vi "LensAndCameraCalibration-GFV.vi"(8 "error in (no error)":errorcluster, 10 "Variant In":variant, 11 "LensCalibrationCtl":T1=enum."Get Calibration") -> (0 "error out":errorcluster, 3 "Variant Out":variant)   [LabVIEW 2015]
doc: "Use this template to build a VI to use as a subVI."
uses:
  LensCalibrationCtlGFV.ctl
  LensCalibrationModel.ctl
  <vilib>/Utility/file.llb/Read From Spreadsheet File (string).vi
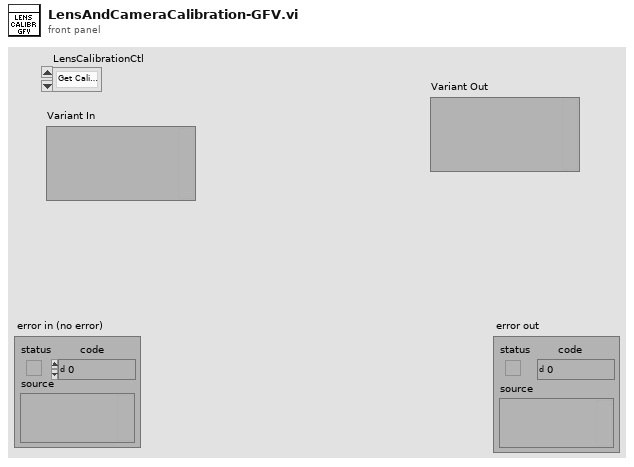
[diagram p1: front panel]
types:
  T1 = typedef "LensCalibrationCtlGFV.ctl" = enum16{"Get MicronPerPixel", "Get Range and PixelsForRange", "Get Mag Names", "Get Calibration", "Read Calibration From File", "Init"}
  T2 = cluster{"MagRingText":u16, "High Resolution":bool}
  T3 = typedef "LensCalibrationModel.ctl" = cluster{"Lens Mag":string, "MicronsPerPixels":dbl, "Scale in microns":i32, "High Resolution":bool}[]
  T4 = cluster{"Lens Mag":string, "MicronsPerPixels":dbl, "Scale in microns":i32, "High Resolution":bool}
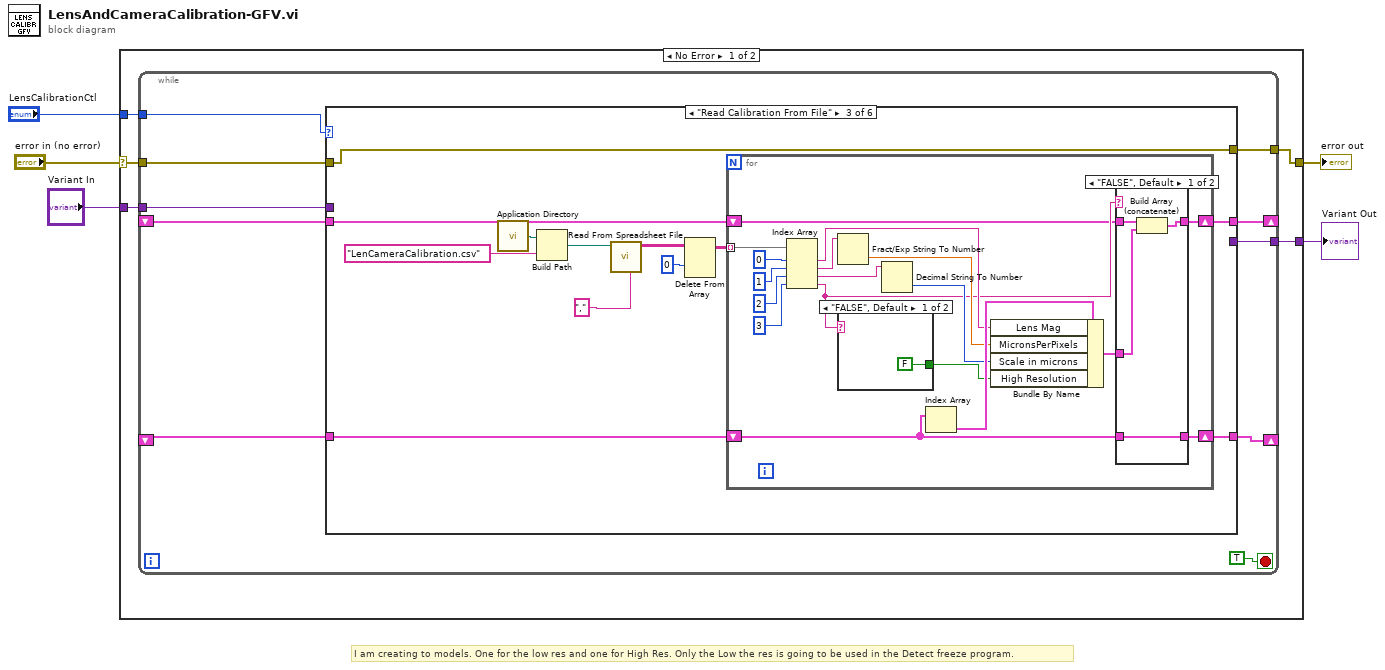
[diagram p0: block diagram]
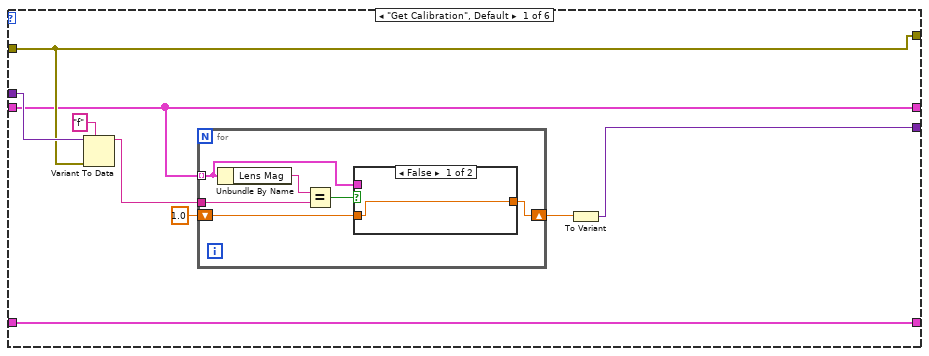
[diagram p2: hidden frame]
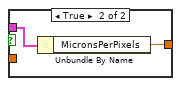
[diagram p3: hidden frame]
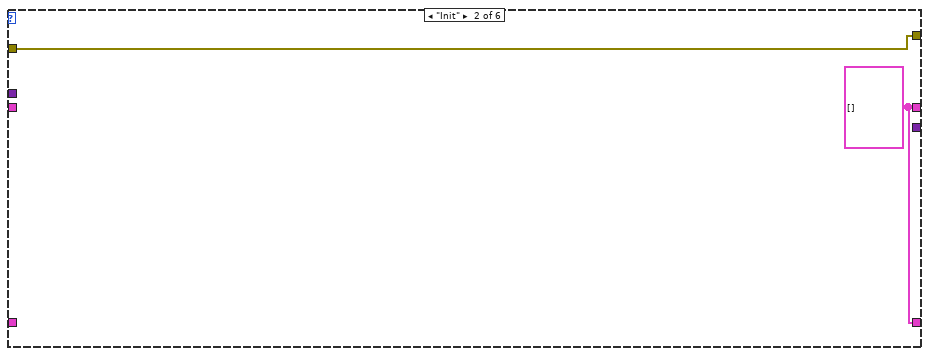
[diagram p4: hidden frame]
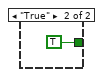
[diagram p5: hidden frame]
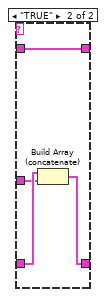
[diagram p6: hidden frame]
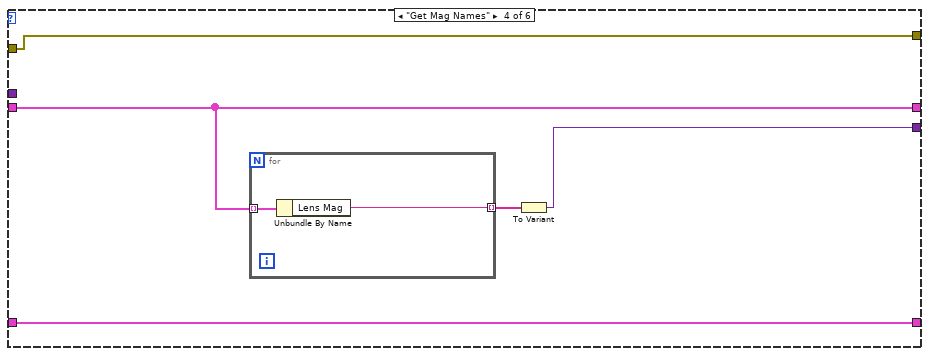
[diagram p7: hidden frame]
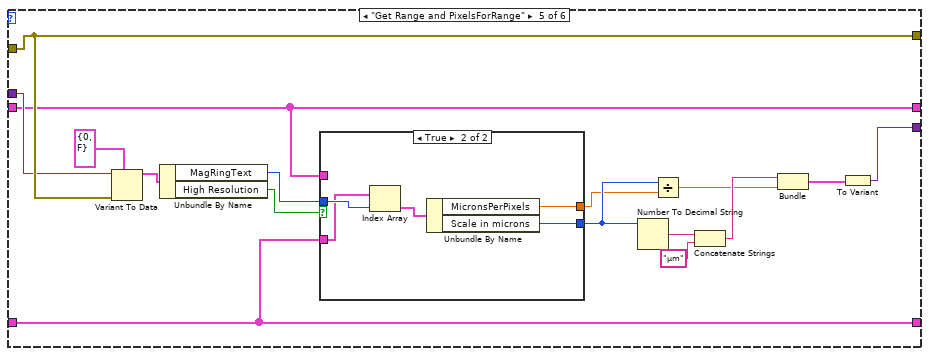
[diagram p8: hidden frame]
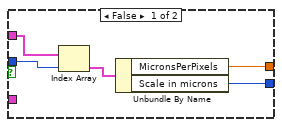
[diagram p9: hidden frame]
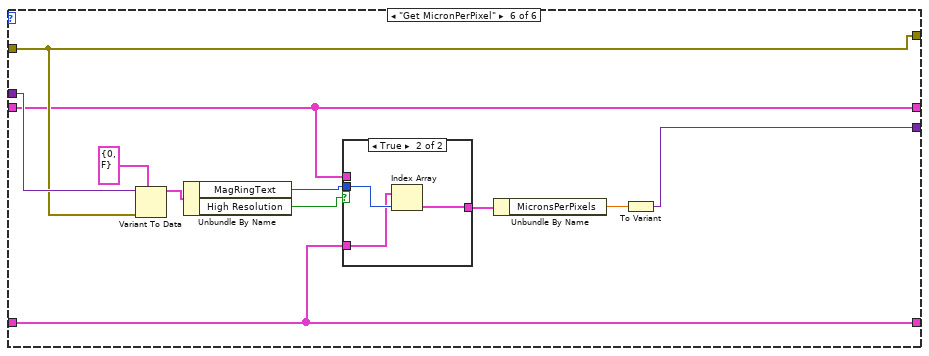
[diagram p10: hidden frame]
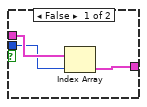
[diagram p11: hidden frame]
diagram:
  # "I am creating to models. One for the low res and one for High Res. Only the Low the res is going to be used in the Detect freeze program."
  n1 = case shown="No Error" "error in (no error)" {
    selector: "error in (no error)" -> [w9 w131]
    tunnel: [w8 w131] -> w4
    tunnel: "LensCalibrationCtl" -> [w10 _]
    tunnel: [w7 _] -> w2
    tunnel: "Variant In" -> [w6 _]
    frame No Error {
      n2 = while {
        tunnel: w10 -> [w19]
        tunnel: w9 -> [w18]
        shift-right: [w14] -> _
        shift-left: _ -> [w15]
        shift-right: [w16] -> _
        shift-left: _ -> [w17]
        tunnel: [w13] -> w8
        tunnel: [w12] -> w7
        tunnel: w6 -> [w11]
        stop <- TRUE stop-if-true
        n3 = case shown="\"Read Calibration From File\"" w19 {
          tunnel: w18 -> [w27 w39 w41 w84 w102 w121]
          tunnel: w17 -> [w29 _ w45 w85 w98 w119]
          tunnel: [w29 w40 w44 w85 w98 w119] -> w16
          tunnel: w15 -> [w25 _ w43 w83 w97 w120]
          tunnel: [w25 w40 w42 w83 w97 w120] -> w14
          tunnel: [w27 w39 w41 w84 w102 w121] -> w13
          tunnel: [w21 _ _ w81 w92 w114] -> w12
          tunnel: w11 -> [w28 _ _ _ w101 w122]
          frame "Get Calibration", Default {
            n4 = Variant To Data(error in=w27, type="f" ("element"), Variant=w28) -> (data=w24:string)  [unwired: 1 out]
            n5 = for {
              tunnel: w25 -> [w32] mode=indexing
              tunnel: w24 -> [w34]
              shift-right: [w31] -> w22
              shift-left: 1.0 ("MicronsPerPixels") -> [w30]
              n6 = Unbundle By Name(w32) -> ("Lens Mag"=w35:string)
              n7 = Equal?(x=w35, y=w34) -> (x = y?=w33:bool)
              n8 = case shown="False" w33 {
                tunnel: w32 -> [_ w38]
                tunnel: [w36 w37] -> w31
                tunnel: w30 -> [w36 _]
                frame False {
                }
                frame True {
                  n9 = Unbundle By Name(w38) -> ("MicronsPerPixels"=w37:dbl)
                }
              }
            }
            n10 = To Variant(anything=w22) -> (Variant=w21:variant)
          }
          frame "Init" {
            w40 = T3 [] ("LensLowRes")
          }
          frame "Read Calibration From File" {
            n11 = call <vilib>:"Application Directory.vi"() -> ("Application Directory"=w49:path)
            n12 = Build Path(base path=w49, name or relative path="LenCameraCalibration.csv") -> (appended path=w47:path)
            n13 = call-poly <vilib>:"Read From Spreadsheet File.vi"("delimiter (\\t)"="," ("delimiter (\\t)"), "file path (dialog if empty)"=w47) -> ("all rows"=w51:string[][])  [unwired: 5 in, 4 out]
            n14 = Delete From Array(array=w51, index (row)=0 ("index")) -> (array with subset deleted=w52:string[][])  [unwired: 2 in, 1 out]
            n15 = for {
              tunnel: w52 -> [w70] mode=indexing
              shift-right: [w53] -> w42
              shift-left: w43 -> [w54]
              shift-right: [w60] -> w44
              shift-left: w45 -> [w62]
              n16 = Index Array(array=w70, index #1=0 ("index"), index #2=1 ("index"), index #3=2 ("index"), index #4=3 ("index")) -> (element #1=w59:string, element #2=w65:string, element #3=w64:string, element #4=w56:string)
              n17 = Fract/Exp String To Number(string=w65) -> (number=w58:dbl)  [unwired: 3 in, 1 out]
              n18 = case shown="\"FALSE\", Default" w56 {
                tunnel: [FALSE TRUE] -> w55
                frame "FALSE", Default {
                }
                frame "True" {
                }
              }
              n19 = Decimal String To Number(string=w64) -> (number=w57:i32)  [unwired: 2 in, 1 out]
              n20 = Index Array(array=w62) -> (element=w63:T4)  [unwired: 1 in]
              n21 = Bundle By Name(cluster=w63, "Lens Mag"=w59, "MicronsPerPixels"=w58, "Scale in microns"=w57, "High Resolution"=w55) -> (w61:T4)
              n22 = case shown="\"FALSE\", Default" w56 {
                tunnel: w62 -> [w73 w80]
                tunnel: w61 -> [w75 w79]
                tunnel: [w73 w78] -> w60
                tunnel: w54 -> [w76 w77]
                tunnel: [w74 w77] -> w53
                frame "FALSE", Default {
                  n23 = Build Array (concatenate)(w76, w75) -> (w74:T3)
                }
                frame "TRUE" {
                  n24 = Build Array (concatenate)(w80, w79) -> (w78:T3)
                }
              }
            }
          }
          frame "Get Mag Names" {
            n25 = for {
              tunnel: w83 -> [w87] mode=indexing
              tunnel: [w86] -> w82 mode=indexing
              n26 = Unbundle By Name(w87) -> ("Lens Mag"=w86:string)
            }
            n27 = To Variant(anything=w82) -> (Variant=w81:variant)
          }
          frame "Get Range and PixelsForRange" {
            n28 = Variant To Data(error in=w102, type=T2 {"MagRingText"=0, "High Resolution"=FALSE} ("output cluster"), Variant=w101) -> (data=w100:T2)  [unwired: 1 out]
            n29 = Unbundle By Name(w100) -> ("MagRingText"=w96:u16, "High Resolution"=w99:bool)
            n30 = case shown="True" w99 {
              tunnel: w98 -> [_ w109]
              tunnel: w97 -> [w107 _]
              tunnel: w96 -> [w108 w113]
              tunnel: [w105 w111] -> w89
              tunnel: [w104 w110] -> w90
              frame False {
                n31 = Index Array(array=w107, index=w108) -> (element=w106:T4)
                n32 = Unbundle By Name(w106) -> ("MicronsPerPixels"=w105:dbl, "Scale in microns"=w104:i32)
              }
              frame True {
                n33 = Index Array(array=w109, index=w113) -> (element=w112:T4)
                n34 = Unbundle By Name(w112) -> ("MicronsPerPixels"=w111:dbl, "Scale in microns"=w110:i32)
              }
            }
            n35 = Number To Decimal String(number=w90) -> (decimal integer string=w95:string)  [unwired: 1 in]
            n36 = Divide(x=w90, y=w89) -> (x/y=w88:dbl)
            n37 = Concatenate Strings(w95, "µm" ("string")) -> (w91:string)
            n38 = Bundle(w91, w88) -> (w93:cluster{string, dbl})  [unwired: 1 in]
            n39 = To Variant(anything=w93) -> (Variant=w92:variant)
          }
          frame "Get MicronPerPixel" {
            n40 = Variant To Data(error in=w121, type=T2 {"MagRingText"=0, "High Resolution"=FALSE} ("output cluster"), Variant=w122) -> (data=w123:T2)  [unwired: 1 out]
            n41 = Unbundle By Name(w123) -> ("MagRingText"=w117:u16, "High Resolution"=w118:bool)
            n42 = case shown="True" w118 {
              tunnel: w120 -> [w127 _]
              tunnel: w119 -> [_ w129]
              tunnel: w117 -> [w126 w130]
              tunnel: [w125 w128] -> w116
              frame False {
                n43 = Index Array(array=w127, index=w126) -> (element=w125:T4)
              }
              frame True {
                n44 = Index Array(array=w129, index=w130) -> (element=w128:T4)
              }
            }
            n45 = Unbundle By Name(w116) -> ("MicronsPerPixels"=w115:dbl)
            n46 = To Variant(anything=w115) -> (Variant=w114:variant)
          }
        }
      }
    }
    frame Error {
    }
  }
  "error out" <- w4
  "Variant Out" <- w2
